vi "Graph Data.vi"(2 "Input":cluster{"X":dbl[], "Y":dbl[]}, 3 "Action":T1) -> (0 "Output":cluster{"X":dbl[], "Y":dbl[]})   [LabVIEW 2013]
uses:
  Action.ctl
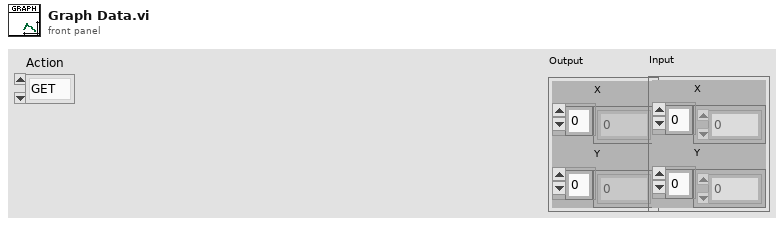
[diagram p1: front panel]
types:
  T1 = typedef "Action.ctl" = enum16{"GET", "PUT", "DELETE"}
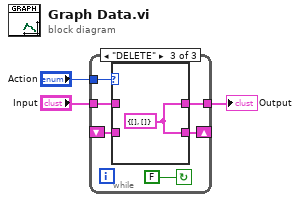
[diagram p0: block diagram]
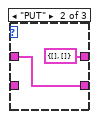
[diagram p3: hidden frame]
diagram:
  n1 = while {
    tunnel: "Action" -> [w8]
    tunnel: [w7] -> w2
    tunnel: "Input" -> [w6]
    shift-right: [w5] -> _
    shift-left: _ -> [w4]
    stop <- FALSE continue-if-true
    n2 = case shown="\"DELETE\"" w8 {
      tunnel: [w10 cluster{"X":dbl[], "Y":dbl[]} {"X"=[], "Y"=[]} ("Input") w13] -> w7
      tunnel: w6 -> [_ w12 _]
      tunnel: [w10 w12 w13] -> w5
      tunnel: w4 -> [w10 _ _]
      frame "GET", Default {
      }
      frame "PUT" {
      }
      frame "DELETE" {
        w13 = cluster{"X":dbl[], "Y":dbl[]} {"X"=[], "Y"=[]} ("Input")
      }
    }
  }
  "Output" <- w2
